vi "GetObjectFromAddress.vi"(8 "error in (no error)":errorcluster, 10 "object address":string, 11 "reference in":refnum<class "Object_Editor.lvclass">) -> (0 "error out":errorcluster, 1 "Ancestor":string, 2 "object":refnum<class "ViPER.lvclass">, 3 "reference out":refnum<class "Object_Editor.lvclass">, 4 "is ancestor":bool, 6 "root object":bool)   [LabVIEW 2022 SP3, in "Object_Editor.lvlib" / "Object_Editor.lvclass"]
uses:
  Object_Editor.lvclass
  Components/ViPER.lvlibp/ViPER.lvclass
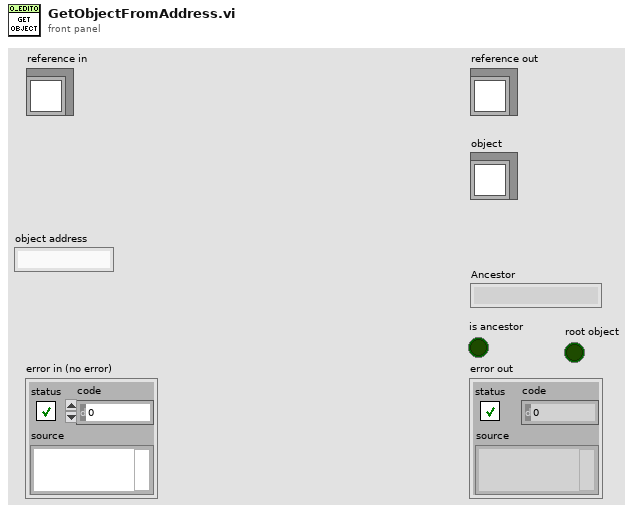
[diagram p1: front panel]
types:
  T1 = typedef "Object_Editor.lvlib/Object_Editor.lvclass/ObjectAttributes.ctl" = cluster{"Config":T2, "Tree":refnum<vi>, "Mod_Bit":bool, "File_Path":path, "Object":refnum<class "ViPER.lvclass">}
  T2 = typedef "Object_Editor.lvlib/Object_Editor.lvclass/Config.ctl" = cluster{"default":string}
  T3 = cluster{"Ancestor":string, "Objects":refnum<class "ViPER.lvclass">[], "Object_Names":string[], "Owned":bool[]}[]
  T4 = cluster{"Ancestor":string, "Objects":refnum<class "ViPER.lvclass">[], "Object_Names":string[], "Owned":bool[]}
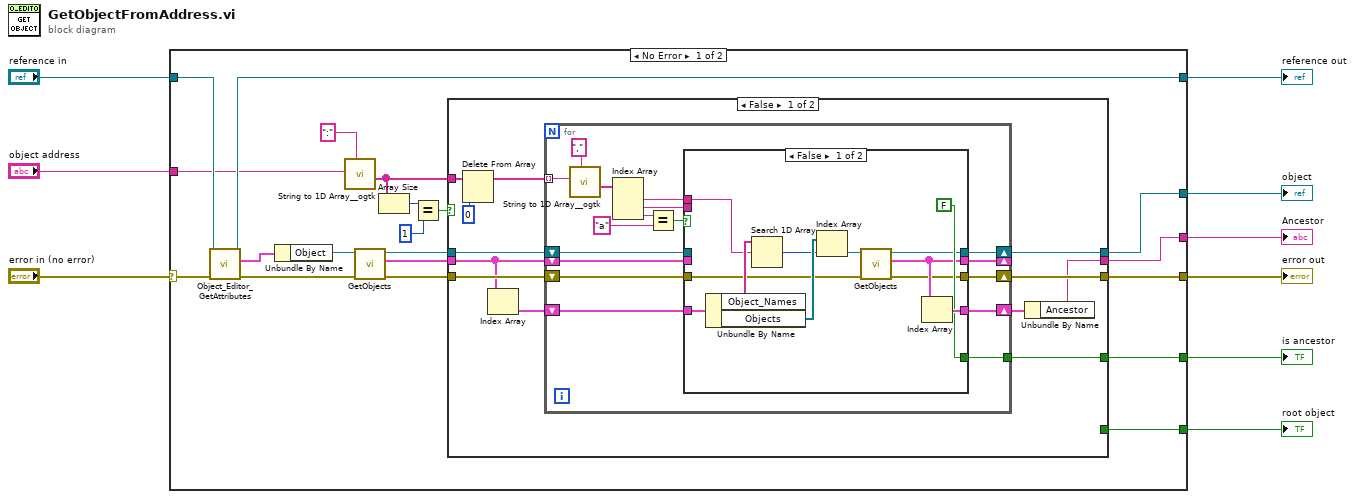
[diagram p0: block diagram]
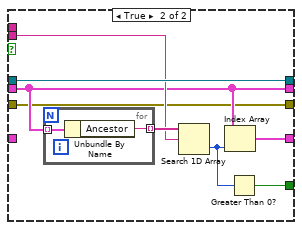
[diagram p2: hidden frame]
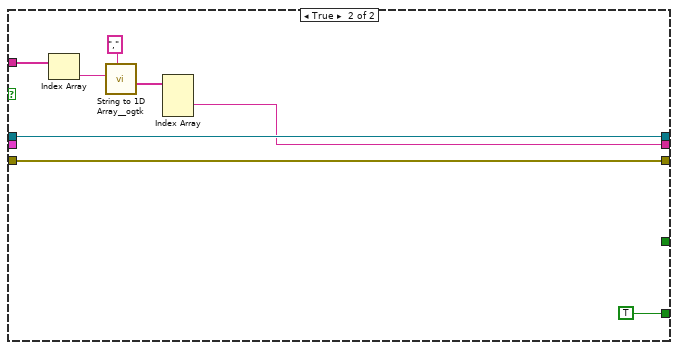
[diagram p3: hidden frame]
diagram:
  n1 = case shown="No Error" "error in (no error)" {
    selector: "error in (no error)" -> [w27 w90]
    tunnel: [w19 w90] -> w8
    tunnel: [w28 w89] -> w6
    tunnel: "reference in" -> [w29 w89]
    tunnel: "object address" -> [w20 _]
    tunnel: [w18 _] -> w1
    tunnel: [w17 _] -> w4
    tunnel: [w16 _] -> w3
    tunnel: [w15 _] -> w2
    frame No Error {
      n2 = call "Object_Editor_GetAttributes.vi"("error in (no error)"=w27, "reference in"=w29) -> ("error out"=w13:errorcluster, "Data"=w26:T1, "reference out"=w28:refnum<class "Object_Editor.lvclass">)  [unwired: 6 in, 1 out]
      n3 = Unbundle By Name(w26) -> ("Object"=w14:refnum<class "ViPER.lvclass">)
      n4 = call <userlib>:"String to 1D Array__ogtk.vi"("delimiter (Tab)"=":", "string"=w20) -> ("Array of Strings"=w24:string[])  [unwired: 9 in]
      n5 = call "GetObjects.vi"("error in (no error)"=w13, "reference in"=w14) -> ("error out"=w10:errorcluster, "Ancestors"=w11:T3, "reference out"=w12:refnum<class "ViPER.lvclass">)  [unwired: 7 in]
      n6 = Array Size(array=w24) -> (size(s)=w23:i32)
      n7 = Equal?(x=w23, y=1) -> (x = y?=w21:bool)
      n8 = case shown="False" w21 {
        tunnel: w10 -> [w41 w87]
        tunnel: w11 -> [w37 _]
        tunnel: w12 -> [w38 w88]
        tunnel: [w35 w88] -> w18
        tunnel: [w34 w87] -> w19
        tunnel: w24 -> [w40 w86]
        tunnel: [w32 w82] -> w17
        tunnel: [w30 _] -> w16
        tunnel: [_ TRUE] -> w15
        frame False {
          n9 = Delete From Array(array=w40, index=0) -> (array with subset deleted=w39:string[])  [unwired: 1 in, 1 out]
          n10 = Index Array(array=w37) -> (element=w36:T4)  [unwired: 1 in]
          n11 = for {
            shift-right: [w43] -> w34
            shift-left: w41 -> [w53]
            shift-right: [w46] -> _
            shift-left: w37 -> [w47]
            tunnel: w39 -> [w57] mode=indexing
            shift-right: [w49] -> w35
            shift-left: w38 -> [w52]
            shift-right: [w45] -> w33
            shift-left: w36 -> [w50]
            tunnel: [w42] -> w30
            n12 = call <userlib>:"String to 1D Array__ogtk.vi"("delimiter (Tab)"=",", "string"=w57) -> ("Array of Strings"=w56:string[])  [unwired: 9 in]
            n13 = Index Array(array=w56) -> (element #1=w44:string, element #2=w48:string, element #3=w55:string)  [unwired: 3 in]
            n14 = Equal?(x=w55, y="a") -> (x = y?=w51:bool)
            n15 = case shown="False" w51 {
              tunnel: w53 -> [w60 w73]
              tunnel: w52 -> [_ w78]
              tunnel: w50 -> [w70 _]
              tunnel: [w62 w78] -> w49
              tunnel: w48 -> [_ w76]
              tunnel: w47 -> [_ w75]
              tunnel: [w61 w75] -> w46
              tunnel: [w65 w74] -> w45
              tunnel: w44 -> [w68 _]
              tunnel: [w59 w73] -> w43
              tunnel: [FALSE w71] -> w42
              frame False {
                n16 = Unbundle By Name(w70) -> ("Object_Names"=w69:string[], "Objects"=w67:refnum<class "ViPER.lvclass">[])
                n17 = Search 1D Array(1D array=w69, element=w68) -> (index of element=w66:i32)  [unwired: 1 in]
                n18 = Index Array(array=w67, index=w66) -> (element=w63:refnum<class "ViPER.lvclass">)
                n19 = call "GetObjects.vi"("error in (no error)"=w60, "reference in"=w63) -> ("error out"=w59:errorcluster, "Ancestors"=w61:T3, "reference out"=w62:refnum<class "ViPER.lvclass">)  [unwired: 7 in]
                n20 = Index Array(array=w61) -> (element=w65:T4)  [unwired: 1 in]
              }
              frame True {
                n21 = for {
                  tunnel: w75 -> [w80] mode=indexing
                  tunnel: [w79] -> w77 mode=indexing
                  n22 = Unbundle By Name(w80) -> ("Ancestor"=w79:string)
                }
                n23 = Search 1D Array(1D array=w77, element=w76) -> (index of element=w72:i32)  [unwired: 1 in]
                n24 = Index Array(array=w75, index=w72) -> (element=w74:T4)
                n25 = Greater Than 0?(x=w72) -> (x > 0?=w71:bool)
              }
            }
          }
          n26 = Unbundle By Name(w33) -> ("Ancestor"=w32:string)
        }
        frame True {
          n27 = Index Array(array=w86) -> (element=w85:string)  [unwired: 1 in]
          n28 = call <userlib>:"String to 1D Array__ogtk.vi"("delimiter (Tab)"=",", "string"=w85) -> ("Array of Strings"=w83:string[])  [unwired: 9 in]
          n29 = Index Array(array=w83) -> (element #2=w82:string)  [unwired: 3 in, 2 out]
        }
      }
    }
    frame Error {
    }
  }
  "error out" <- w8
  "reference out" <- w6
  "Ancestor" <- w4
  "is ancestor" <- w3
  "root object" <- w2
  "object" <- w1
